vi "Heise Barometric Pressure 901A Main.vi"(8 "Error In":errorcluster, 11 "VISA Refnum in":refnum<visa-resource-name>) -> (0 "Error Out":errorcluster)   [LabVIEW 2016]
panel:
  out "Barometric Data":string[](array[string])
  in  "stop":bool
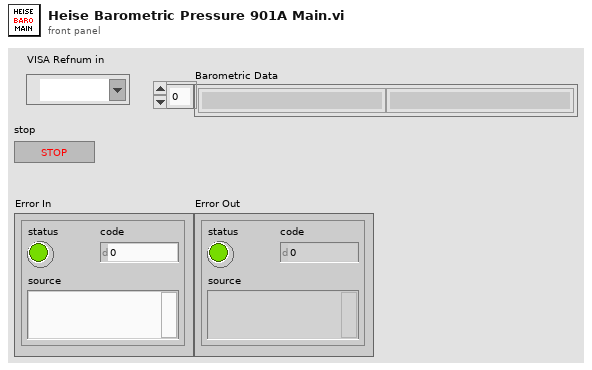
[diagram p1: front panel]
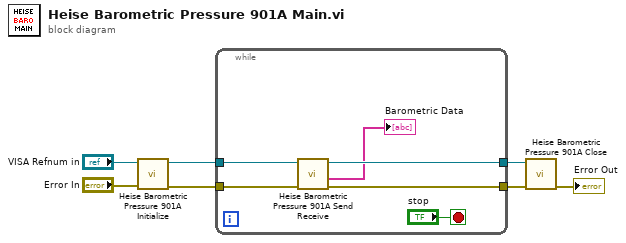
[diagram p0: block diagram]
diagram:
  n1 = call "Heise Barometric Pressure 901A Initialize.vi"("error in (no error)"="Error In", "VISA Refnum in"="VISA Refnum in") -> ("error out"=w3:errorcluster, "VISA Refnum out"=w4:refnum<visa-resource-name>)  [unwired: 8 in]
  n2 = while {
    tunnel: [w12] -> w7
    tunnel: [w11] -> w6
    tunnel: w4 -> [w10]
    tunnel: w3 -> [w9]
    stop <- "stop" stop-if-true
    n3 = call "Heise Barometric Pressure 901A Send Receive.vi"("error in (no error)"=w9, "VISA Refnum in"=w10) -> ("error out"=w11:errorcluster, "Barometric Data"=→"Barometric Data":string[], "VISA Refnum out"=w12:refnum<visa-resource-name>)  [unwired: 6 in, 1 out]
  }
  n4 = call "Heise Barometric Pressure 901A Close.vi"("error in (no error)"=w6, "VISA Refnum in"=w7) -> ("error out"=→"Error Out":errorcluster)  [unwired: 9 in]
